vi "main.vi"(7 "Last Experiment of the Day":bool, 8 "error in":errorcluster, 9 "SSH password":string, 10 "SSH user name":string, 11 "Tags":string) -> (0 "error out":errorcluster)   [LabVIEW 2019]
uses:
  WormTrackSnippetCluster.ctl
  TrackTerminationReasonEnum.ctl
  HeadTailContinuousGWN.lvclass
  C:/github/ProjectAPI/LabviewVIs/StimulusObject.lvclass
  HeadTailContinuousGWNClass/HeadTailContinuousGWNInputCluster.ctl
  <vilib>/vision/driver/IMAQdx.llb/IMAQdx Acquisition Mode.ctl
  CompletedTracksFunctionalGlobalOperations.ctl
  ActiveTracksFunctionalGlobalOperations.ctl
  TimestampsFunctionalGlobalOperations.ctl
  <vilib>/vision/driver/IMAQdx.llb/IMAQdx Buffer Number Mode.ctl
  center2rectangle.vi
  overlay_crossmarks.vi
  ParametersGlobal.vi
  DebugGlobal.vi
  <vilib>/vision/driver/NI_Vision_Acquisition_Software.lvlib
  <vilib>/vision/NI_Vision_Development_Module.lvlib
panel:
  out "Experiment Start":dbl
  out "Spatial Correction Fit Error (camera pixel)":dbl
  out "transformation_description":dbl[](array[numeric])
  out "Latest Active Worm Tracks":T1[](array[typedef])
  out "Mature Tracks Count":i32
  out "Active Tracks Count":i32
  out "total time elapsed (s)":dbl
  out "Draw Stimulus Missed Frames":dbl
  out "Tracking Missed Frames":dbl
  out "Camera Missed Frames":dbl
  out "Last Calibration":dbl
  in  "GUI Refresh Period (ms)":u32=10000
  out "Stop Debug":string
  out "Completed Tracks #":i32
  out "Projector Saving Lag (Projector Frames)":i32
  out "Stimulus Image":T3(plugin-control)
  out "Closed Loop Lag (frames)":i32
  out "Single Worm Image":T3(plugin-control)
  in  "Selected Track Index":i32
  out "Tracking Rate (Hz)":dbl
  out "Last Median Filter Updated":string
  out "median closed loop lag (ms)":dbl
  out "Draw Stimulus Frame Rate (Hz)":dbl
  out "Saving Lag (Camera Frames)":i32
  out "Camera Frame Rate (Hz)":dbl
  out "Camera Buffer Number":u32
  in  "stop":bool
  out "Camera Input":T3(plugin-control)
  out "Processed Image":T3(plugin-control)
  # "Max Spatial Drift (mm) Since:"
  # "Guide to spatial re-alignment Processed Image:\nPink circles represents previous calibration locations.\nAqua circle means the calibration for this iteration.\nYellow lines show deviation from previous calibration loation to locations extracted just now.\nMagenta lines at the end shows drift since the experiment began"
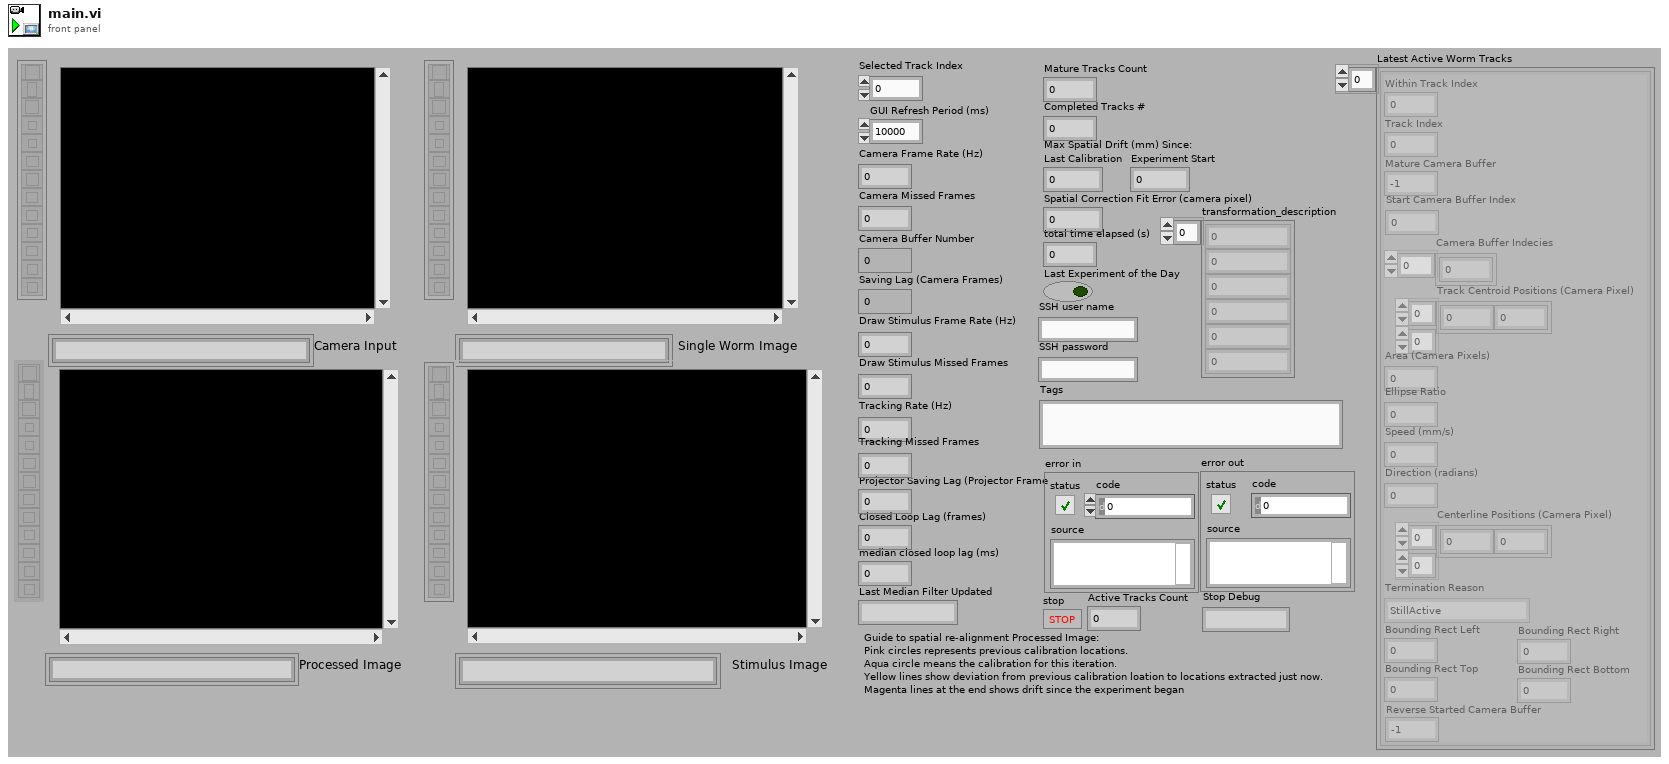
[diagram p1: front panel]
types:
  T1 = typedef "WormTrackSnippetCluster.ctl" = cluster{"Track Centroid Positions (Camera Pixel)":sgl[][], "Within Track Index":i32, "Camera Buffer Indecies":i32[], "Area (Camera Pixels)":i32, "Speed (mm/s)":sgl, "Direction (radians)":sgl, "Centerline Positions (Camera Pixel)":sgl[][], "Ellipse Ratio":sgl, "Termination Reason":T2, "Track Index":i32, "Bounding Rect Left":i32, "Bounding Rect Top":i32, "Bounding Rect Right":i32, "Bounding Rect Bottom":i32, "Mature Camera Buffer":i32, "Start Camera Buffer Index":i32, "Reverse Started Camera Buffer":i32}
  T2 = typedef "TrackTerminationReasonEnum.ctl" = enum16{"StillActive", "MaxDisplacement", "NoBlobsLeft", "AreaIncrease", "AreaDecrease", "ExperimentEnded"}
  T3 = typedef "IMAQ Image.ctl" = refnum<image>
  T4 = typedef "HeadTailContinuousGWN.lvclass/HeadTailContinuousGWNInputCluster.ctl" = cluster{"offset (red uW/mm^2m, blue is negative)":sgl, "correlation time (s)":sgl, "standard deviation (red uW/mm^2)":sgl, "Max blue stimulus (uW/mm^2)":sgl, "Max red stimulus (uW/mm^2)":sgl, "dot radius (mm)":sgl}
  T5 = typedef "TimestampsFunctionalGlobalOperations.ctl" = enum16{"Initialize", "Dump", "UpdateTime", "ReadTime"}
  T6 = typedef "ActiveTracksFunctionalGlobalOperations.ctl" = enum16{"Initialize", "ReadFullTrackGivenWormIndex", "WriteFullTrack", "ReadTrackSnippets", "WriteTrackGivenSnippets", "ReadStimulusSnippets", "StartNewTracksGivenSnippets", "EndTracksGivenSnippets", "WriteStimulusObjectGivenWormIndex", "CompleteAllActiveTracks", "ReturnAllActiveTrackIndecies"}
  T7 = typedef "CompletedTracksFunctionalGlobalOperations.ctl" = enum16{"Initialize", "ReturnAllTracks", "ReturnLastIndex", "SaveCompletedTracks", "TrimAndReturnAllTracks"}
  T8 = typedef "NI_Vision_Acquisition_Software.lvlib/IMAQdx Buffer Number Mode.ctl" = enum32{"Next", "Last", "Buffer Number", "Every", "Last New"}
  T9 = typedef "Image Type" = u32
  T10 = typedef "NI_Vision_Acquisition_Software.lvlib/IMAQdx Acquisition Mode.ctl" = enum32{"One Shot", "Continuous"}
  T11 = typedef "IMAQdx.ctl" = refnum<k21>
  T12 = typedef "WormTrackCluster.ctl" = cluster{"Track Centroid Positions (Camera Pixel)":sgl[][], "Within Track Index":i32, "Camera Buffer Indecies":i32[], "Area (Camera Pixels)":i32[], "Speed (mm/s)":sgl[], "Direction (radians)":sgl[], "Centerline Positions (Camera Pixel)":sgl[][][], "Ellipse Ratio":sgl[], "Stimulus Object":refnum<class "StimulusObject.lvclass">, "Termination Reason":T2, "Track Index":i32, "Mature Camera Buffer":i32, "Reverse Started Camera Buffer":i32}
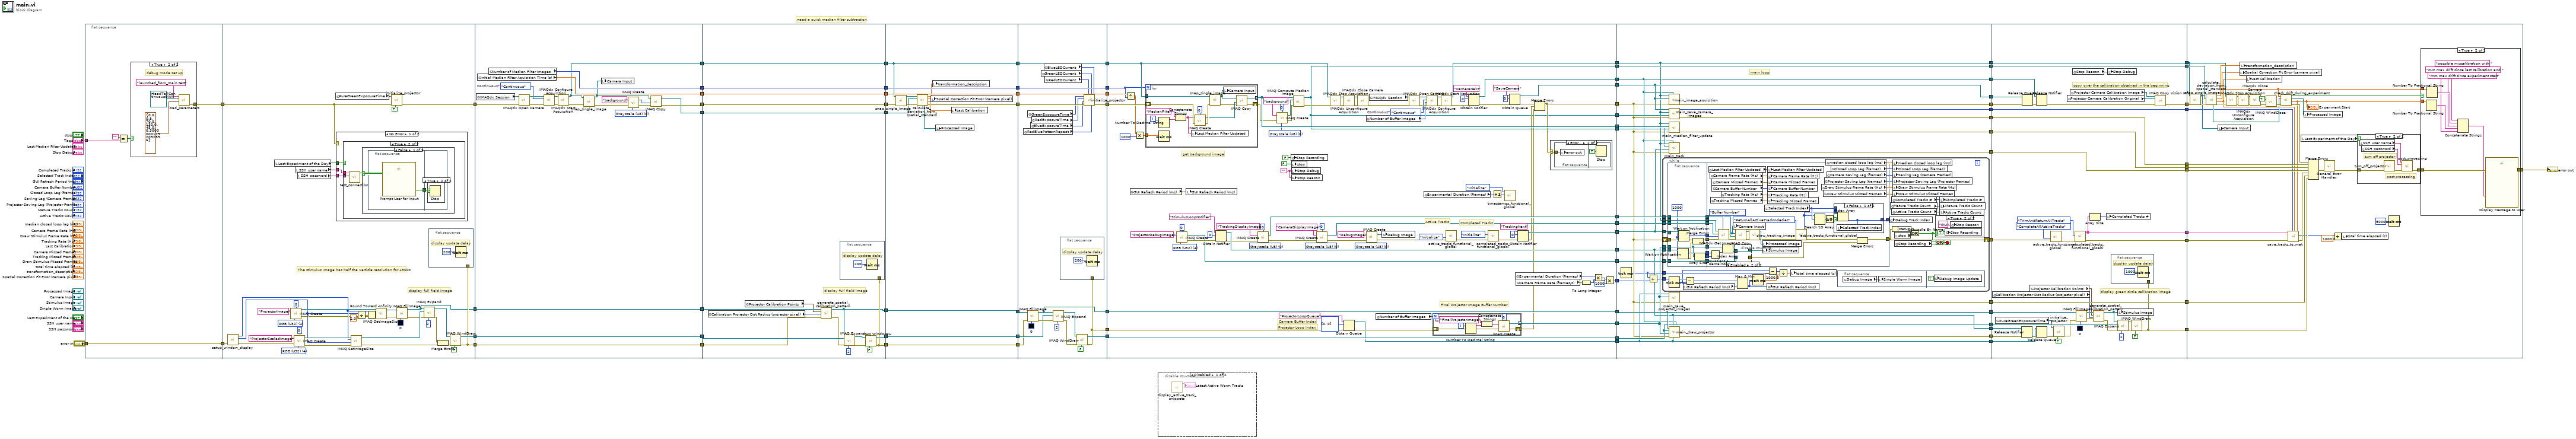
[diagram p0: block diagram]
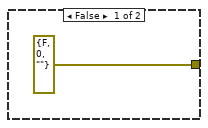
[diagram p3: hidden frame]
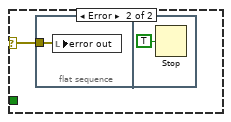
[diagram p7: hidden frame]
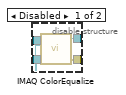
[diagram p11: hidden frame]
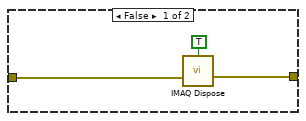
[diagram p12: hidden frame]
diagram:
  # "need a quick median filter subtraction"
  n1 = flat-sequence {
    tunnel: "Tags" -> [w85]
    tunnel: "error in" -> [w89]
    tunnel: [w89] -> w28
    tunnel: [w86] -> w27
    tunnel: [w125] -> w77
    tunnel: [w104] -> w76
    tunnel: [w99] -> w75
    tunnel: [w97] -> w63
    tunnel: w28 -> [w113]
    tunnel: w27 -> [w98]
    tunnel: [w148] -> w20
    tunnel: w77 -> [w157]
    tunnel: w76 -> [w158]
    tunnel: [w158] -> w21
    tunnel: [w154] -> w22
    tunnel: w75 -> [w156]
    tunnel: [w167] -> w23
    tunnel: [w166] -> w24
    tunnel: w63 -> [w160]
    tunnel: [w157] -> w25
    tunnel: [w156] -> w26
    tunnel: [w147] -> w4
    tunnel: w26 -> [w173]
    tunnel: [w168] -> w19
    tunnel: w25 -> [w179]
    tunnel: [w178] -> w17
    tunnel: w24 -> [w185]
    tunnel: [w185] -> w15
    tunnel: w23 -> [w184]
    tunnel: [w184] -> w13
    tunnel: w22 -> [w183]
    tunnel: [w183] -> w11
    tunnel: w21 -> [w174]
    tunnel: [w175] -> w9
    tunnel: w20 -> [w182]
    tunnel: [w182] -> w7
    tunnel: [w176] -> w5
    tunnel: w4 -> [w176]
    tunnel: w19 -> [w201]
    tunnel: [w201] -> w18
    tunnel: w17 -> [w200]
    tunnel: [w200] -> w16
    tunnel: w15 -> [w199]
    tunnel: [w199] -> w14
    tunnel: w13 -> [w198]
    tunnel: [w198] -> w12
    tunnel: w11 -> [w193]
    tunnel: [w193] -> w10
    tunnel: w9 -> [w197]
    tunnel: [w197] -> w8
    tunnel: w7 -> [w195]
    tunnel: [w187] -> w6
    tunnel: w5 -> [w191]
    tunnel: [w209] -> w35
    tunnel: [w225] -> w34
    tunnel: [w224] -> w33
    tunnel: [w223] -> w32
    tunnel: [w222] -> w31
    tunnel: [w221] -> w30
    tunnel: [w220] -> w29
    tunnel: w18 -> [w214]
    tunnel: w16 -> [w213]
    tunnel: w14 -> [w220]
    tunnel: w12 -> [w221]
    tunnel: w10 -> [w223]
    tunnel: w8 -> [w212]
    tunnel: w6 -> [w210]
    tunnel: [w303] -> w84
    tunnel: [w252] -> w83
    tunnel: [w291] -> w82
    tunnel: [w240] -> w81
    tunnel: w35 -> [w316]
    tunnel: w34 -> [w303]
    tunnel: w33 -> [w246]
    tunnel: w32 -> [w263]
    tunnel: w31 -> [w291]
    tunnel: [w227] -> w80
    tunnel: [w312] -> w79
    tunnel: [w311] -> w78
    tunnel: [w308] -> w74
    tunnel: [w292] -> w73
    tunnel: [w286] -> w72
    tunnel: [w283] -> w71
    tunnel: [w278] -> w70
    tunnel: [w275] -> w69
    tunnel: [w268] -> w68
    tunnel: w30 -> [w251]
    tunnel: w29 -> [w250]
    tunnel: [w227] -> w64
    tunnel: [w227] -> w62
    tunnel: [w244] -> w37
    tunnel: [w236] -> w36
    tunnel: [w372] -> w61
    tunnel: w84 -> [w357]
    tunnel: w83 -> [w352]
    tunnel: w82 -> [w358]
    tunnel: w81 -> [w348]
    tunnel: [w353] -> w60
    tunnel: [w371] -> w59
    tunnel: [w370] -> w58
    tunnel: [w352] -> w56
    tunnel: w80 -> [w351]
    tunnel: w79 -> [w368]
    tunnel: [w369] -> w54
    tunnel: w78 -> [w353]
    tunnel: w74 -> [w349]
    tunnel: [w349] -> w52
    tunnel: [w367] -> w51
    tunnel: w73 -> [w366]
    tunnel: [w365] -> w49
    tunnel: w72 -> [w355]
    tunnel: w71 -> [w354]
    tunnel: w70 -> [w356]
    tunnel: w69 -> [w364]
    tunnel: w68 -> [w363]
    tunnel: [w362] -> w48
    tunnel: [w356] -> w46
    tunnel: w64 -> [w361]
    tunnel: [w360] -> w45
    tunnel: w62 -> [w359]
    tunnel: [w359] -> w44
    tunnel: [w357] -> w40
    tunnel: [w358] -> w39
    tunnel: [w354] -> w38
    tunnel: w37 -> [w350]
    tunnel: w36 -> [w346]
    tunnel: w61 -> [w505]
    tunnel: w60 -> [w513]
    tunnel: w59 -> [w511]
    tunnel: w58 -> [w520]
    tunnel: [w520] -> w57
    tunnel: w56 -> [w519]
    tunnel: [w519] -> w55
    tunnel: w54 -> [w518]
    tunnel: [w518] -> w53
    tunnel: w52 -> [w512]
    tunnel: w51 -> [w517]
    tunnel: [w517] -> w50
    tunnel: w49 -> [w507]
    tunnel: w48 -> [w516]
    tunnel: [w516] -> w47
    tunnel: w46 -> [w504]
    tunnel: w45 -> [w482]
    tunnel: w44 -> [w515]
    tunnel: [w515] -> w43
    tunnel: [w485] -> w42
    tunnel: [w492] -> w41
    tunnel: w40 -> [w499]
    tunnel: w39 -> [w495]
    tunnel: w38 -> [w493]
    tunnel: [w482] -> w3
    tunnel: [w481] -> w2
    tunnel: [w480] -> w1
    tunnel: w57 -> [w553]
    tunnel: w55 -> [w538]
    tunnel: w53 -> [w555]
    tunnel: w50 -> [w556]
    tunnel: w47 -> [w554]
    tunnel: [w548] -> w66
    tunnel: w43 -> [w541]
    tunnel: w42 -> [w542]
    tunnel: w41 -> [w547]
    tunnel: w3 -> [w528]
    tunnel: w2 -> [w527]
    tunnel: w1 -> [w526]
    frame #0 {
      n2 = Equal?(x="", y=w85) -> (x = y?=w88:bool)
      n3 = case shown="True" w88 {
        tunnel: [errorcluster {"status"=FALSE, "code"=0, "source"=""} ("error in") w94] -> w86
        frame False {
        }
        frame True {
          # "debug mode set up"
          n4 = call "load_parameters.vi"("StimulusObject Parameters"=T4 {"offset (red uW/mm^2m, blue is negative)"=0.0, "correlation time (s)"=0.5, "standard deviation (red uW/mm^2)"=70.0, "Max blue stimulus (uW/mm^2)"=130.0, "Max red stimulus (uW/mm^2)"=45.0, "dot radius (mm)"=0.3} ("HeadTailContinousGWNInputCluser"), "StimulusObjectClassInput"=refnum<class "HeadTailContinuousGWN.lvclass"> refnum ("HeadTailContinuousGWN.lvclass"), "Tags"="launched_from_main test") -> ("error out"=w94:errorcluster)  [unwired: 6 in, 2 out]
        }
      }
    }
    frame #1 {
      w123 = T9 4 items=["Grayscale (U8)", "Grayscale (I16)", "Grayscale (SGL)", "Complex (CSG)", "RGB (U32)", "HSL (U32)", "RGB (U64)"] ("Image Type")
      w127 = T9 4 items=["Grayscale (U8)", "Grayscale (I16)", "Grayscale (SGL)", "Complex (CSG)", "RGB (U32)", "HSL (U32)", "RGB (U64)"] ("Image Type")
      # "The stimulus Image has half the verticle resolution for 4500s"
      # "display full field image"
      n5 = call "setup_window_display.vi"("error in (no error)"=w113) -> ("error out"=w130:errorcluster, "Height"=w117:i16, "Width"=w121:i16)  [unwired: 8 in]
      n6 = local read "Last Experiment of the Day"() -> (w110:bool)
      n7 = call "IMAQ Create"("Border Size"=0, "Image Name"="ProjectorImage", "Image Type"=w123) -> ("New Image"=w122:T3, "error out"=w116:errorcluster)  [unwired: 2 in]
      n8 = call "IMAQ Create"("Border Size"=0, "Image Name"="ProjectorScaledImage", "Image Type"=w127, "error in (no error)"=w130) -> ("New Image"=w131:T3, "error out"=w132:errorcluster)  [unwired: 1 in]
      n9 = local read "SSH user name"() -> (w111:string)
      n10 = local read "SSH password"() -> (w112:string)
      n11 = global read "ParametersGlobal.vi" "PureGreenExposureTime"() -> (w95:i32)
      n12 = case shown="No Error" w98 {
        selector: w98 -> [_ w143]
        tunnel: w112 -> [w136 _]
        tunnel: w111 -> [w135 _]
        tunnel: w110 -> [w134 _]
        frame No Error {
          n13 = case shown="True" w134 {
            tunnel: w136 -> [_ w139]
            tunnel: w135 -> [_ w137]
            frame False {
            }
            frame True {
              n14 = call "test_connection.vi"("Username"=w137, "Password"=w139) -> ("Connection Successful"=w138:bool)  [unwired: 7 in]
              n15 = case shown="False" w138 {
                frame False {
                  n16 = flat-sequence {
                    tunnel: [w141] -> w140
                    tunnel: w140 -> [w142]
                    frame #0 {
                      n17 = call "Prompt User for Input"() -> ("OK"=w141:bool)  [unwired: 18 in, 1 out]
                    }
                    frame #1 {
                      n18 = case shown="True" w142 {
                        frame False {
                        }
                        frame True {
                          n19 = Stop() -> ()  [unwired: 1 in]
                        }
                      }
                    }
                  }
                }
                frame True {
                }
              }
            }
          }
        }
        frame Error {
          n20 = flat-sequence {
            tunnel: w143 -> [w144]
            frame #0 {
              n21 = local write "error out"(w144) -> ()
            }
            frame #1 {
              n22 = Stop(stop? (T)=TRUE) -> ()
            }
          }
        }
      }
      n23 = call "IMAQ SetImageSize"("error in (no error)"=w132, "Y Resolution"=w117, "X Resolution"=w121, "Image"=w131) -> ("error out"=w105:errorcluster, "Image Out"=w108:T3)  [unwired: 1 in]
      n24 = Divide(x=w117, y=2.0) -> (x/y=w119:dbl)
      n25 = Round Toward -Infinity(1:w119) -> (0:w120:dbl)
      n26 = call "IMAQ SetImageSize"("error in (no error)"=w116, "Y Resolution"=w120, "X Resolution"=w121, "Image"=w122) -> ("error out"=w102:errorcluster, "Image Out"=w100:T3)  [unwired: 1 in]
      n27 = call "initialize_projector.vi"("Green Only"=TRUE, "error in"=w98, "green exp_time_us"=w95) -> ("error out"=w97:errorcluster)  [unwired: 8 in]
      n28 = call "IMAQ FillImage"("Color Pixel Value"=u32 0, "error in (no error)"=w102, "Image"=w100) -> ("error out"=w101:errorcluster, "Image Out"=w99:T3)  [unwired: 7 in]
      n29 = call "IMAQ Expand"("Y Duplication Step"=2, "error in (no error)"=w101, "Image Dst"=w108, "Image Src"=w99) -> ("error out"=w106:errorcluster, "Image Dst Out"=w107:T3)  [unwired: 6 in]
      n30 = flat-sequence {
        tunnel: w104 -> [_]
        frame #0 {
          # "display update delay"
          n31 = Wait (ms)(milliseconds to wait=u32 200) -> ()  [unwired: 1 out]
        }
      }
      n32 = Merge Errors(w106, w105) -> (w115:errorcluster)
      n33 = call "IMAQ WindDraw"("Resize to Image Size? (Y)"=FALSE, "error in (no error)"=w115, "Image"=w107) -> ("error out"=w104:errorcluster, "Image Out (duplicate)"=w125:T3)  [unwired: 7 in]
    }
    frame #2 {
      w146 = T9 0 items=["Grayscale (U8)", "Grayscale (I16)", "Grayscale (SGL)", "Complex (CSG)", "RGB (U32)", "HSL (U32)", "RGB (U64)", "Grayscale (U16)"] ("Image Type")
      w159 = IMAQdx_Acquisition_Mode."Continuous"  # Continuous?
      n34 = global read "ParametersGlobal.vi" "IMAQdx Session"() -> (w165:T11)
      n35 = global read "ParametersGlobal.vi" "Initial Median Filter Aquisition Time (s)"() -> (w167:dbl)
      n36 = global read "ParametersGlobal.vi" "Number of Median Filter Images"() -> (w166:i32)
      n37 = call <vilib>:"IMAQdx Open Camera.vi"("error in"=w160, "Session In"=w165) -> ("error out"=w162:errorcluster, "Session Out"=w161:T11)  [unwired: 8 in]
      n38 = call <vilib>:"IMAQdx Configure Acquisition.vi"("error in"=w162, "Continuous?"=w159, "Session In"=w161) -> ("error out"=w163:errorcluster, "Session Out"=w164:T11)  [unwired: 7 in]
      n39 = call <vilib>:"IMAQdx Start Acquisition.vi"("error in"=w163, "Session In"=w164) -> ("error out"=w155:errorcluster, "Session Out"=w154:T11)  [unwired: 8 in]
      n40 = call "snap_single_image.vi"("error in (no error)"=w155, "Session In"=w154) -> ("error out"=w152:errorcluster, "Image Out"=w149:T3)  [unwired: 8 in]
      n41 = local write "Camera Input"(w149) -> ()
      n42 = call "IMAQ Create"("Image Name"="background", "Image Type"=w146, "error in (no error)"=w152) -> ("New Image"=w150:T3, "error out"=w151:errorcluster)  [unwired: 2 in]
      n43 = call "IMAQ Copy"("error in (no error)"=w151, "Image Dst"=w150, "Image Src"=w149) -> ("error out"=w148:errorcluster, "Image Dst Out"=w147:T3)  [unwired: 3 in]
    }
    frame #3 {
      # "display full field image"
      n44 = global read "ParametersGlobal.vi" "Calibration Projector Dot Radius (projector pixel)"() -> (w171:i32)
      n45 = global read "ParametersGlobal.vi" "Projector Calibration Points"() -> (w170:cluster{"X":dbl, "Y":dbl}[])
      n46 = call "generate_spatial_calibration_pattern.vi"("error in (no error)"=w174, "Dot Radius (Projector Pixels)"=w171, "Points Array"=w170, "StimulusImageIn"=w173) -> ("error out"=w172:errorcluster, "StimulusImageOut"=w168:T3)  [unwired: 6 in]
      n47 = flat-sequence {
        tunnel: w175 -> [_]
        frame #0 {
          # "display update delay"
          n48 = Wait (ms)(milliseconds to wait=u32 200) -> ()  [unwired: 1 out]
        }
      }
      n49 = call "IMAQ Expand"("Y Duplication Step"=2, "error in (no error)"=w172, "Image Dst"=w179, "Image Src"=w168) -> ("error out"=w177:errorcluster, "Image Dst Out"=w169:T3)  [unwired: 6 in]
      n50 = call "IMAQ WindDraw"("Resize to Image Size? (Y)"=FALSE, "error in (no error)"=w177, "Image"=w169) -> ("error out"=w175:errorcluster, "Image Out (duplicate)"=w178:T3)  [unwired: 7 in]
    }
    frame #4 {
      n51 = call "snap_single_image.vi"("error in (no error)"=w195, "Session In"=w193) -> ("error out"=w194:errorcluster, "Image Out"=w192:T3)  [unwired: 8 in]
      n52 = call "calculate_deviation_from_spatial_standard.vi"("Image Src"=w192, "Background Image"=w191, "error in (no error)"=w194) -> ("Processed Image"=w188:T3, "transformation_description"=w196:dbl[], "fit least squares error (camera pixel)"=w189:dbl, "max spatial drift (mm)"=w190:dbl, "error out"=w187:errorcluster)  [unwired: 3 in]
      n53 = local write "Spatial Correction Fit Error (camera pixel)"(w189) -> ()
      n54 = local write "transformation_description"(w196) -> ()
      n55 = local write "Processed Image"(w188) -> ()
      n56 = local write "Last Calibration"(w190) -> ()
    }
    frame #5 {
      n57 = global read "ParametersGlobal.vi" "RedBluePatternRepeat"() -> (w202:i32)
      n58 = call "IMAQ FillImage"("Color Pixel Value"=u32 0, "error in (no error)"=w212, "Image"=w214) -> ("error out"=w219:errorcluster, "Image Out"=w222:T3)  [unwired: 7 in]
      n59 = global read "ParametersGlobal.vi" "GreenExposureTime"() -> (w205:i32)
      n60 = global read "ParametersGlobal.vi" "BlueExposureTime"() -> (w203:i32)
      n61 = global read "ParametersGlobal.vi" "RedExposureTime"() -> (w204:i32)
      n62 = global read "ParametersGlobal.vi" "GreenLEDCurrent"() -> (w207:u8)
      n63 = global read "ParametersGlobal.vi" "BlueLEDCurrent"() -> (w206:u8)
      n64 = global read "ParametersGlobal.vi" "RedLEDCurrent"() -> (w208:u8)
      n65 = call "IMAQ Expand"("Y Duplication Step"=2, "error in (no error)"=w219, "Image Dst"=w213, "Image Src"=w222) -> ("error out"=w215:errorcluster, "Image Dst Out"=w211:T3)  [unwired: 6 in]
      n66 = flat-sequence {
        tunnel: w224 -> [_]
        frame #0 {
          # "display update delay"
          n67 = Wait (ms)(milliseconds to wait=u32 200) -> ()  [unwired: 1 out]
        }
      }
      n68 = call "IMAQ WindDraw"("Resize to Image Size? (Y)"=FALSE, "error in (no error)"=w215, "Image"=w211) -> ("error out"=w224:errorcluster, "Image Out (duplicate)"=w225:T3)  [unwired: 7 in]
      n69 = call "initialize_projector.vi"("BlueCurrent"=w206, "RedBluePatternRepeat"=w202, "GreenCurrent"=w207, "RedCurrent"=w208, "error in"=w210, "blue exp_time_us"=w203, "red exp_time_us"=w204, "green exp_time_us"=w205) -> ("error out"=w209:errorcluster)  [unwired: 3 in]
    }
    frame #6 {
      w229 = T9 0 items=["Grayscale (U8)", "Grayscale (I16)", "Grayscale (SGL)", "Complex (CSG)", "RGB (U32)", "HSL (U32)", "RGB (U64)", "Grayscale (U16)"] ("Image Type")
      w258 = IMAQdx_Acquisition_Mode."Continuous"  # Continuous?
      w247 = ""
      w272 = T9 0 items=["Grayscale (U8)", "Grayscale (I16)", "Grayscale (SGL)", "Complex (CSG)", "RGB (U32)", "HSL (U32)", "RGB (U64)", "Grayscale (U16)"] ("Image Type")
      w282 = T9 4 items=["Grayscale (U8)", "Grayscale (I16)", "Grayscale (SGL)", "Complex (CSG)", "RGB (U32)", "HSL (U32)", "RGB (U64)", "Grayscale (U16)"] ("Image Type")
      w296 = T9 0 items=["Grayscale (U8)", "Grayscale (I16)", "Grayscale (SGL)", "Complex (CSG)", "RGB (U32)", "HSL (U32)", "RGB (U64)", "Grayscale (U16)"] ("Image Type")
      w301 = T9 0 items=["Grayscale (U8)", "Grayscale (I16)", "Grayscale (SGL)", "Complex (CSG)", "RGB (U32)", "HSL (U32)", "RGB (U64)", "Grayscale (U16)"] ("Image Type")
      # "Projector Loop Index"
      # "Camera Buffer Index"
      # "Final Projector Image Buffer Number"
      # "Active Tracks"
      # "Completed Tracks"
      # "get background image"
      n70 = Divide(x=w251, y=w250) -> (x/y=w307:dbl)
      n71 = global read "DebugGlobal.vi" "GUI Refresh Period (ms)"() -> (w233:u32)
      n72 = Multiply(x=w307, y=1000) -> (x*y=w305:dbl)
      n73 = for {
        N: w250 -> [_]
        tunnel: w263 -> [w344]
        shift-right: [w333] -> w302
        shift-left: w316 -> [w340]
        tunnel: [w336] -> w312 mode=indexing
        tunnel: w305 -> [w335]
        i -> [w343]
        n74 = Wait (ms)(milliseconds to wait=w335) -> ()  [unwired: 1 out]
        n75 = Number To Decimal String(number=w343) -> (decimal integer string=w342:string)  [unwired: 1 in]
        n76 = Concatenate Strings("MedianFilter", w342) -> (w331:string)
        n77 = local write "Last Median Filter Updated"(w331) -> ()
        n78 = call "IMAQ Create"("Border Size"=0, "Image Name"=w331, "error in (no error)"=w340) -> ("New Image"=w338:T3, "error out"=w339:errorcluster)  [unwired: 2 in]
        n79 = call "snap_single_image.vi"("error in (no error)"=w339, "Session In"=w344) -> ("error out"=w337:errorcluster, "Image Out"=w332:T3)  [unwired: 8 in]
        n80 = local write "Camera Input"(w332) -> ()
        n81 = call "IMAQ Copy"("error in (no error)"=w337, "Image Dst"=w338, "Image Src"=w332) -> ("error out"=w333:errorcluster, "Image Dst Out"=w336:T3)  [unwired: 3 in]
      }
      n82 = call "IMAQ Create"("Border Size"=0, "Image Name"="ProjectorDebugImage", "Image Type"=w282) -> ("New Image"=w275:T3, "error out"=w276:errorcluster)  [unwired: 2 in]
      n83 = local write "GUI Refresh Period (ms)"(w233) -> ()
      n84 = Obtain Notifier(name (unnamed)="StimulusLoopNotifier", notification data type=0, error in (no error)=w276) -> (notifier out=w278:refnum<notifier>, error out=w270:errorcluster)  [unwired: 1 in, 1 out]
      n85 = call "IMAQ Create"("Border Size"=0, "Image Name"="TrackingDisplayImage", "Image Type"=w272, "error in (no error)"=w270) -> ("New Image"=w268:T3, "error out"=w269:errorcluster)  [unwired: 1 in]
      n86 = call "IMAQ Create"("Border Size"=0, "Image Name"="background", "Image Type"=w229, "error in (no error)"=w302) -> ("New Image"=w313:T3, "error out"=w314:errorcluster)  [unwired: 1 in]
      n87 = global write "DebugGlobal.vi" "Stop Recording"(FALSE ("Stop Recording")) -> ()
      n88 = local write "stop"(FALSE) -> ()
      n89 = local write "Stop Debug"(w247) -> ()
      n90 = global write "DebugGlobal.vi" "Stop Reason"(w247) -> ()
      n91 = call "IMAQ Compute Median Image"("error in (no error)"=w314, "Image Dst"=w313, "Images"=w312) -> ("error out"=w228:errorcluster, "Image Dst Out"=w227:T3)  [unwired: 7 in]
      n92 = call "IMAQ Create"("Border Size"=0, "Image Name"="CameraDisplayImage", "Image Type"=w296, "error in (no error)"=w269) -> ("New Image"=w292:T3, "error out"=w293:errorcluster)  [unwired: 1 in]
      n93 = call <vilib>:"IMAQdx Stop Acquisition.vi"("error in"=w228, "Session In"=w263) -> ("error out"=w264:errorcluster, "Session Out"=w265:T11)  [unwired: 8 in]
      n94 = call <vilib>:"IMAQdx Unconfigure Acquisition.vi"("error in"=w264, "Session In"=w265) -> ("error out"=w267:errorcluster, "Session Out"=w266:T11)  [unwired: 8 in]
      n95 = Obtain Queue(name (unnamed)="ProjectorLoopQueue", element data type=i32[] [0, 0], error in (no error)=w246) -> (queue out=w283:refnum<queue>, error out=w284:errorcluster)  [unwired: 2 in, 1 out]
      n96 = call <vilib>:"IMAQdx Close Camera.vi"("error in"=w267, "Session In"=w266) -> ("error out"=w256:errorcluster)  [unwired: 9 in]
      n97 = global read "ParametersGlobal.vi" "Number of Buffer Images"() -> (w254:i32)
      n98 = call "IMAQ Create"("Image Name"="DebugImage", "Image Type"=w301, "error in (no error)"=w293) -> ("New Image"=w299:T3, "error out"=w245:errorcluster)  [unwired: 2 in]
      n99 = global read "ParametersGlobal.vi" "IMAQdx Session"() -> (w257:T11)
      n100 = global read "ParametersGlobal.vi" "Number of Buffer Images"() -> (w253:i32)
      n101 = global write "DebugGlobal.vi" "Debug Image"(w299) -> ()
      n102 = call <vilib>:"IMAQdx Open Camera.vi"("error in"=w256, "Session In"=w257) -> ("error out"=w261:errorcluster, "Session Out"=w262:T11)  [unwired: 8 in]
      n103 = global read "ParametersGlobal.vi" "Experimental Duration (Frames)"() -> (w232:i32)
      n104 = call <vilib>:"IMAQdx Configure Acquisition.vi"("error in"=w261, "Number of Buffers"=w254, "Continuous?"=w258, "Session In"=w262) -> ("error out"=w260:errorcluster, "Session Out"=w259:T11)  [unwired: 6 in]
      n105 = for {
        N: w253 -> [_]
        shift-right: [w324] -> w241
        shift-left: w284 -> [w327]
        tunnel: [w323] -> w286 mode=indexing
        i -> [w330]
        n106 = Number To Decimal String(number=w330) -> (decimal integer string=w329:string)  [unwired: 1 in]
        n107 = Concatenate Strings("FinalProjectorImage", w329) -> (w326:string)
        n108 = call "IMAQ Create"("Border Size"=0, "Image Name"=w326, "error in (no error)"=w327) -> ("New Image"=w323:T3, "error out"=w324:errorcluster)  [unwired: 2 in]
      }
      n109 = call <vilib>:"IMAQdx Start Acquisition.vi"("error in"=w260, "Session In"=w259) -> ("error out"=w255:errorcluster, "Session Out"=w252:T11)  [unwired: 8 in]
      n110 = call "active_tracks_functional_global.vi"("error in"=w245, "Operations"=ActiveTracksFunctionalGlobalOperations."Initialize") -> ("error out"=w288:errorcluster)  [unwired: 5 in, 4 out]
      n111 = Obtain Notifier(name (unnamed)="CameraNext", notification data type=u32 0, error in (no error)=w255) -> (notifier out=w308:refnum<notifier>, error out=w249:errorcluster)  [unwired: 1 in, 1 out]
      n112 = call "completed_tracks_functional_gloabl.vi"("error in (no error)"=w288, 10:CompletedTracksFunctionalGlobalOperations."Initialize") -> ("error out"=w289:errorcluster)  [unwired: 6 in, 3 out]
      n113 = Increment(x=w232) -> (x+1=w231:i32)
      n114 = call "timestamps_functional_global.vi"("Buffer Number"=w231, "Operation"=TimestampsFunctionalGlobalOperations."Initialize") -> ()  [unwired: 3 in, 3 out]
      n115 = Obtain Queue(name (unnamed)="SaveCamera", element data type=u32 0, error in (no error)=w249) -> (queue out=w311:refnum<queue>, error out=w243:errorcluster)  [unwired: 2 in, 1 out]
      n116 = global read "ParametersGlobal.vi" "Experimental Duration (Frames)"() -> (w239:i32)
      n117 = global read "ParametersGlobal.vi" "Camera Frame Rate (frames/s)"() -> (w235:sgl)
      n118 = Obtain Notifier(name (unnamed)="TrackingNext", notification data type=u32 0, error in (no error)=w289) -> (notifier out=w244:refnum<notifier>, error out=w242:errorcluster)  [unwired: 1 in, 1 out]
      n119 = Merge Errors(w243, w242, w241) -> (w240:errorcluster)
      n120 = case shown="Error .." w240 {
        selector: w240 -> [_ w320]
        frame No Error {
        }
        frame Error {
          n121 = flat-sequence {
            tunnel: w320 -> [w321]
            frame #0 {
              n122 = local write "error out"(w321) -> ()
            }
            frame #1 {
              n123 = Stop(stop? (T)=TRUE) -> ()
            }
          }
        }
      }
      n124 = To Long Integer(number=w235) -> (32bit integer=w234:i32)
      n125 = Multiply(x=w239, y=w234) -> (x*y=w238:i32)
      n126 = Multiply(x=w238, y=1000) -> (x*y=w236:i32)
    }
    frame #7 {
      # "main loop"
      n127 = Tick Count (ms)() -> (millisecond timer value=w347:u32)
      n128 = Add(x=w347, y=w346) -> (x+y=w345:u32)
      n129 = while {
        shift-right: [w406] -> w365
        shift-left: w348 -> [w413]
        tunnel: w350 -> [w414]
        tunnel: w352 -> [w410]
        tunnel: w366 -> [w407]
        tunnel: w356 -> [w404]
        tunnel: w355 -> [w402]
        tunnel: w364 -> [w400]
        tunnel: w363 -> [w397]
        tunnel: w347 -> [w387]
        tunnel: w345 -> [w382]
        stop <- w390 stop-if-true
        n130 = flat-sequence {
          tunnel: w414 -> [w433]
          tunnel: w413 -> [w432]
          tunnel: [w426] -> w412
          tunnel: [w431] -> w411
          tunnel: w410 -> [w430]
          tunnel: [w430] -> w409
          tunnel: [w429] -> w408
          tunnel: w407 -> [w429]
          tunnel: w404 -> [w428]
          tunnel: [w427] -> w403
          tunnel: w402 -> [w419]
          tunnel: [w419] -> w401
          tunnel: w400 -> [w423]
          tunnel: [w423] -> w399
          tunnel: [w422] -> w398
          tunnel: w397 -> [w422]
          tunnel: [w420] -> w388
          tunnel: w412 -> [w466]
          tunnel: [w452] -> w406
          tunnel: w411 -> [w465]
          tunnel: w409 -> [w464]
          tunnel: w408 -> [w463]
          tunnel: w403 -> [w462]
          tunnel: w401 -> [w461]
          tunnel: w399 -> [w459]
          tunnel: w398 -> [w456]
          tunnel: w388 -> [w443]
          tunnel: [w436] -> w375
          frame #0 {
            w421 = 1000 ("timeout in ms (-1)")
            n131 = Wait on Notification(notifier=w428, timeout in ms (-1)=w421) -> (notification=w427:i32, error out=w424:errorcluster)  [unwired: 2 in, 2 out]
            n132 = Wait on Notification(notifier=w433, timeout in ms (-1)=w421, error in (no error)=w432) -> (notification=w431:u32, error out=w425:errorcluster)  [unwired: 1 in, 2 out]
            n133 = Merge Errors(w425, w424) -> (w426:errorcluster)
            n134 = Array Size(array=w419) -> (size(s)=w420:i32)
          }
          frame #1 {
            n135 = global read "DebugGlobal.vi" "Last Median Filter Updated"() -> (w444:string)
            n136 = global read "DebugGlobal.vi" "Camera Frame Rate (Hz)"() -> (w447:dbl)
            n137 = Quotient & Remainder(x=w462, y=w443) -> (x-y*floor(x/y)=w442:i32)  [unwired: 1 out]
            n138 = global read "DebugGlobal.vi" "Tracking Missed Frames"() -> (w445:dbl)
            n139 = global read "DebugGlobal.vi" "Camera Buffer Number"() -> (w448:u32)
            n140 = global read "DebugGlobal.vi" "Camera Missed Frames"() -> (w446:dbl)
            n141 = call <vilib>:"IMAQdx Get Image.vi"("Buffer Number Mode (Next)"=IMAQdx_Buffer_Number_Mode."Buffer Number", "error in"=w466, "Buffer Number In"=w465, "Image In"=w463, "Session In"=w464) -> ("error out"=w458:errorcluster, "Image Out"=w457:T3)  [unwired: 3 in, 2 out]
            n142 = global read "DebugGlobal.vi" "Tracking Rate (Hz)"() -> (w449:dbl)
            n143 = Index Array(array=w461, index=w442) -> (element=w460:T3)
            n144 = local write "Camera Input"(w457) -> ()
            n145 = disable-structure shown="Enabled" {
              disable-tunnel: w460 -> [w474 w475]
              disable-tunnel: w459 -> [w473 _]
              disable-tunnel: [w472 _] -> w451
              disable-tunnel: [w471 w475] -> w450
              frame Disabled {
                n146 = call "IMAQ ColorEqualize"("Image Dst"=w473, "Image Src"=w474) -> ("error out"=w472:errorcluster, "Image Dst Out"=w471:T3)  [unwired: 3 in]
              }
              frame Enabled {
              }
            }
            n147 = call "IMAQ Copy"("error in (no error)"=w458, "Image Dst"=w456, "Image Src"=w457) -> ("error out"=w455:errorcluster, "Image Dst Out"=w454:T3)  [unwired: 3 in]
            n148 = call "draw_tracking_image.vi"("error in (no error)"=w455, "Image In"=w454) -> ("error out"=w435:errorcluster, "Image Out"=w453:T3)  [unwired: 8 in]
            n149 = local write "Processed Image"(w453) -> ()
            n150 = local write "Stimulus Image"(w450) -> ()
            n151 = local read "Selected Track Index"() -> (w438:i32)
            n152 = local write "Last Median Filter Updated"(w444) -> ()
            n153 = local write "Camera Frame Rate (Hz)"(w447) -> ()
            n154 = local write "Camera Missed Frames"(w446) -> ()
            n155 = local write "Camera Buffer Number"(w448) -> ()
            n156 = local write "Tracking Rate (Hz)"(w449) -> ()
            n157 = local write "Tracking Missed Frames"(w445) -> ()
            n158 = call "active_tracks_functional_global.vi"("error in"=w435, "Operations"=ActiveTracksFunctionalGlobalOperations."ReturnAllActiveTrackIndecies") -> ("error out"=w434:errorcluster, "Active Track Indecies"=w437:i32[])  [unwired: 5 in, 3 out]
            n159 = Search 1D Array(1D array=w437, element=w438) -> (index of element=w440:i32)  [unwired: 1 in]
            n160 = Greater Or Equal To 0?(x=w440) -> (x >= 0?=w439:bool)
            n161 = case shown="False" w439 {
              tunnel: w438 -> [_ w470]
              tunnel: w437 -> [w469 _]
              tunnel: [w468 w470] -> w436
              frame False {
                n162 = Index Array(array=w469) -> (element=w468:i32)  [unwired: 1 in]
                n163 = local write "Selected Track Index"(w468) -> ()
              }
              frame True {
              }
            }
            n164 = Merge Errors(w434, w451) -> (w452:errorcluster)
          }
        }
        n165 = Tick Count (ms)() -> (millisecond timer value=w380:u32)
        n166 = local read "GUI Refresh Period (ms)"() -> (w383:u32)
        n167 = Subtract(x=w382, y=w380) -> (x-y=w381:u32)
        n168 = Max & Min(x=w381, y=w383) -> (min(x,y)=w379:u32)  [unwired: 1 out]
        n169 = Wait (ms)(milliseconds to wait=w379) -> ()  [unwired: 1 out]
        n170 = global write "DebugGlobal.vi" "GUI Refresh Period (ms)"(w379) -> ()
        n171 = Subtract(x=w380, y=w387) -> (x-y=w386:u32)
        n172 = Divide(x=w386, y=1000.0) -> (x/y=w384:dbl)
        n173 = local write "total time elapsed (s)"(w384) -> ()
        n174 = global read "DebugGlobal.vi" "Draw Stimulus Frame Rate (Hz)"() -> (w391:dbl)
        n175 = global read "DebugGlobal.vi" "Draw Stimulus Missed Frames"() -> (w392:dbl)
        n176 = global read "DebugGlobal.vi" "Projector Saving Lag (frames)"() -> (w389:i32)
        n177 = global read "DebugGlobal.vi" "median closed loop lag (ms)"() -> (w395:dbl)
        n178 = global read "DebugGlobal.vi" "Camera Saving Lag (frames)"() -> (w393:i32)
        n179 = global read "DebugGlobal.vi" "Closed Loop Lag (frames)"() -> (w394:i32)
        n180 = flat-sequence {
          frame #0 {
            n181 = global read "DebugGlobal.vi" "Debug Image"() -> (w415:T3)
            n182 = local write "Single Worm Image"(w415) -> ()
          }
          frame #1 {
            n183 = global write "DebugGlobal.vi" "Debug Image Update"(TRUE ("Debug Image Update")) -> ()
          }
        }
        n184 = global write "DebugGlobal.vi" "Debug Track Index"(w375) -> ()
        n185 = global read "DebugGlobal.vi" "Mature Tracks Count"() -> (w377:i32)
        n186 = global read "DebugGlobal.vi" "Completed Tracks #"() -> (w376:i32)
        n187 = global read "DebugGlobal.vi" "Active Tracks Count"() -> (w378:i32)
        n188 = Unbundle By Name(w406) -> ("status"=w396:bool)
        n189 = local write "median closed loop lag (ms)"(w395) -> ()
        n190 = local write "Closed Loop Lag (frames)"(w394) -> ()
        n191 = local write "Saving Lag (Camera Frames)"(w393) -> ()
        n192 = local write "Projector Saving Lag (Projector Frames)"(w389) -> ()
        n193 = local write "Draw Stimulus Frame Rate (Hz)"(w391) -> ()
        n194 = local write "Draw Stimulus Missed Frames"(w392) -> ()
        n195 = local read "stop"() -> (w405:bool)
        n196 = global read "DebugGlobal.vi" "Stop Recording"() -> (w374:bool)
        n197 = Or(x=w396, y=w405) -> (x .or. y?=w373:bool)
        n198 = Or(x=w373, y=w374) -> (x .or. y?=w390:bool)
        n199 = case shown="True" w373 {
          frame False {
          }
          frame True {
            n200 = global write "DebugGlobal.vi" "Stop Recording"(TRUE ("stop")) -> ()
            n201 = global write "DebugGlobal.vi" "Stop Reason"("GUI" ("Stop Debug")) -> ()
          }
        }
        n202 = local write "Mature Tracks Count"(w377) -> ()
        n203 = local write "Completed Tracks #"(w376) -> ()
        n204 = local write "Active Tracks Count"(w378) -> ()
      }
      n205 = call "main_image_aquisition.vi"("notifier in"=w349, "error in (no error)"=w348, "queue in"=w353, "Session In"=w352) -> ("error out"=w371:errorcluster)  [unwired: 5 in]
      n206 = call "main_save_camera_images.vi"("error in (no error)"=w348, "Median Filtered Image"=w361, "Session In"=w352, "Queue in"=w353) -> ("error out"=w370:errorcluster, "Decoded Camera Frmes"=w360:i32[])  [unwired: 6 in]
      n207 = call "main_median_filter_update.vi"("error in (no error)"=w348, "Median Filtered Image"=w351, "Spaced Out Images"=w368, "Session In"=w352) -> ("error out"=w369:errorcluster)  [unwired: 7 in]
      n208 = call "main_track.vi"("camera notifier"=w349, "error in (no error)"=w348, "tracking notifier in"=w350, "Median Filter Image"=w351, "Session In"=w352) -> ("error out"=w367:errorcluster)  [unwired: 6 in]
      n209 = call "main_save_projector_images.vi"("error in"=w348, "Array"=w355, "Queue in"=w354) -> ("error out"=w362:errorcluster)  [unwired: 8 in]
      n210 = call "main_draw_projector.vi"("camera notifier in"=w349, "projector loop queue in"=w354, "stimulus loop notifier in"=w356, "error in"=w348, "stimulus saving buffer"=w355, "ProjectorScaledImage in"=w357, "ProjectorImage in"=w358) -> ("error out"=w372:errorcluster)  [unwired: 4 in]
    }
    frame #8 {
      # "copy over the calibration obtained in the beginning"
      # "display green circle calibration image"
      n211 = global read "ParametersGlobal.vi" "Calibration Projector Dot Radius (projector pixel)"() -> (w488:i32)
      n212 = global read "ParametersGlobal.vi" "PureGreenExposureTime"() -> (w476:i32)
      n213 = Release Notifier(notifier=w504, error in (no error)=w505) -> (error out=w506:errorcluster)  [unwired: 1 in, 2 out]
      n214 = Release Queue(queue=w513, error in (no error)=w511) -> (error out=w514:errorcluster)  [unwired: 1 in, 2 out]
      n215 = global read "ParametersGlobal.vi" "Projector Calibration Points"() -> (w487:cluster{"X":dbl, "Y":dbl}[])
      n216 = Release Notifier(notifier=w512, error in (no error)=w514) -> (error out=w486:errorcluster)  [unwired: 1 in, 2 out]
      n217 = Release Queue(queue=w493, error in (no error)=w506) -> (error out=w479:errorcluster)  [unwired: 1 in, 2 out]
      n218 = call "active_tracks_functional_global.vi"("error in"=w507, "Operations"=ActiveTracksFunctionalGlobalOperations."CompleteAllActiveTracks") -> ("error out"=w510:errorcluster)  [unwired: 5 in, 4 out]
      n219 = call "initialize_projector.vi"("Green Only"=TRUE, "error in"=w479, "green exp_time_us"=w476) -> ("error out"=w478:errorcluster)  [unwired: 8 in]
      n220 = global read "ParametersGlobal.vi" "Projector Camera Calibration Original"() -> (w484:T3)
      n221 = global read "ParametersGlobal.vi" "Projector Camera Calibration Image"() -> (w483:T3)
      n222 = global read "DebugGlobal.vi" "Stop Reason"() -> (w494:string)
      n223 = call "completed_tracks_functional_gloabl.vi"("error in (no error)"=w510, 10:CompletedTracksFunctionalGlobalOperations."TrimAndReturnAllTracks") -> ("error out"=w480:errorcluster, "OutputTracks"=w481:T12[])  [unwired: 6 in, 2 out]
      n224 = call "IMAQ FillImage"("Color Pixel Value"=u32 0, "error in (no error)"=w478, "Image"=w495) -> ("error out"=w496:errorcluster, "Image Out"=w490:T3)  [unwired: 7 in]
      n225 = Array Size(array=w481) -> (size(s)=w491:i32)
      n226 = call "generate_spatial_calibration_pattern.vi"("error in (no error)"=w496, "Dot Radius (Projector Pixels)"=w488, "Points Array"=w487, "StimulusImageIn"=w490) -> ("error out"=w502:errorcluster, "StimulusImageOut"=w489:T3)  [unwired: 6 in]
      n227 = local write "Completed Tracks #"(w491) -> ()
      n228 = local write "Stop Debug"(w494) -> ()
      n229 = flat-sequence {
        tunnel: w492 -> [_]
        frame #0 {
          # "display update delay"
          n230 = Wait (ms)(milliseconds to wait=u32 1000) -> ()  [unwired: 1 out]
        }
      }
      n231 = call "IMAQ Expand"("Y Duplication Step"=2, "error in (no error)"=w502, "Image Dst"=w499, "Image Src"=w489) -> ("error out"=w500:errorcluster, "Image Dst Out"=w498:T3)  [unwired: 6 in]
      n232 = local write "Stimulus Image"(w489) -> ()
      n233 = call "IMAQ WindDraw"("Resize to Image Size? (Y)"=FALSE, "error in (no error)"=w500, "Image"=w498) -> ("error out"=w492:errorcluster)  [unwired: 7 in, 1 out]
      n234 = call "IMAQ Copy Vision Info"("error in (no error)"=w486, "Image Dst"=w484, "Image Src"=w483) -> ("error out"=w485:errorcluster)  [unwired: 6 in, 2 out]
    }
    frame #9 {
      n235 = call "snap_single_image.vi"("error in (no error)"=w542, "Session In"=w538) -> ("error out"=w540:errorcluster, "Image Out"=w539:T3)  [unwired: 8 in]
      n236 = call "calculate_deviation_from_spatial_standard.vi"("Image Src"=w539, "Background Image"=w541, "error in (no error)"=w540) -> ("Processed Image"=w533:T3, "transformation_description"=w543:dbl[], "fit least squares error (camera pixel)"=w537:dbl, "max spatial drift (mm)"=w523:dbl, "error out"=w536:errorcluster)  [unwired: 3 in]
      n237 = local write "Camera Input"(w539) -> ()
      n238 = call <vilib>:"IMAQdx Stop Acquisition.vi"("error in"=w536, "Session In"=w538) -> ("error out"=w557:errorcluster, "Session Out"=w558:T11)  [unwired: 8 in]
      n239 = call <vilib>:"IMAQdx Unconfigure Acquisition.vi"("error in"=w557, "Session In"=w558) -> ("error out"=w560:errorcluster, "Session Out"=w559:T11)  [unwired: 8 in]
      n240 = local write "Spatial Correction Fit Error (camera pixel)"(w537) -> ()
      n241 = local write "transformation_description"(w543) -> ()
      n242 = local write "Last Calibration"(w523) -> ()
      n243 = call <vilib>:"IMAQdx Close Camera.vi"("error in"=w560, "Session In"=w559) -> ("error out"=w545:errorcluster)  [unwired: 9 in]
      n244 = call "IMAQ WindClose"("Close All Windows (False)"=TRUE, "error in (no error)"=w545) -> ("error out"=w535:errorcluster)  [unwired: 4 in]
      n245 = call "check_drift_during_experiment.vi"("error in (no error)"=w535, "Processed Image"=w533, "max spatial drift since calibration (mm)"=w523) -> ("error out"=w534:errorcluster, "max spatial drift since experiment start (mm)"=w522:sgl, "Image Out"=w532:T3, "Warning needed"=w550:bool)  [unwired: 5 in]
      "Experiment Start" <- w522
      n246 = call "save_tracks_to_mat.vi"("Max Spatial Drift Since Experiment Start (mm)"=w522, "Max Spatial Drift Since Last Calibration (mm)"=w523, "DecodedCameraFrames"=w528, "error in"=w526, "Completed Tracks"=w527) -> ("error out"=w525:errorcluster, "total time elapsed (ms)"=w524:i32)  [unwired: 4 in, 1 out]
      n247 = local read "Last Experiment of the Day"() -> (w551:bool)
      n248 = local write "Processed Image"(w532) -> ()
      n249 = Merge Errors(w534, w553, w555, w556, w525, w554, w547) -> (w544:errorcluster)
      n250 = call <vilib>:"General Error Handler.vi"("error in (no error)"=w544) -> ("error out"=w552:errorcluster)  [unwired: 10 in, 4 out]
      n251 = Divide(x=w524, y=1000.0) -> (x/y=w530:dbl)
      n252 = local write "total time elapsed (s)"(w530) -> ()
      n253 = case shown="True" w551 {
        tunnel: w552 -> [w574 w576]
        tunnel: [w574 w579] -> w549
        frame False {
        }
        frame True {
          # "turn off projector"
          # "post processing"
          n254 = local read "SSH user name"() -> (w577:string)
          n255 = local read "SSH password"() -> (w578:string)
          n256 = call "turn_off_projector.vi"("error in"=w576) -> ("error out"=w575:errorcluster)  [unwired: 10 in]
          n257 = call "post_processing.vi"("error in (no error)"=w575, "SSH password"=w578, "SSH user name"=w577) -> ("error out"=w579:errorcluster)  [unwired: 8 in]
        }
      }
      n258 = Wait (ms)(milliseconds to wait=u32 5000) -> ()  [unwired: 1 out]
      n259 = case shown="True" w550 {
        tunnel: w549 -> [w562 w573]
        tunnel: [w561 w572] -> w548
        tunnel: w523 -> [_ w571]
        tunnel: w522 -> [_ w570]
        frame False {
          n260 = call "IMAQ Dispose"("All Images? (No)"=TRUE, "error in (no error)"=w562) -> ("error out"=w561:errorcluster)  [unwired: 4 in]
        }
        frame True {
          n261 = Number To Fractional String(number=w570) -> (F-format string=w566:string)  [unwired: 3 in]
          n262 = Number To Fractional String(number=w571) -> (F-format string=w568:string)  [unwired: 3 in]
          n263 = Concatenate Strings("possible miscalibration with ", w568, "mm max drift since last calibration and " ("string"), w566, "mm max drift since experiment start" ("string")) -> (w564:string)
          n264 = call "Display Message to User"("error in (no error)"=w573, "Message"=w564) -> ("error out"=w572:errorcluster)  [unwired: 8 in, 1 out]
        }
      }
    }
  }
  n265 = disable-structure shown="Disabled" {
    frame Disabled {
      n266 = call "display_active_track_snippets.vi"() -> ("Latest Active Worm Tracks"=→"Latest Active Worm Tracks":T1[])  [unwired: 3 in, 3 out]
    }
    frame Enabled {
    }
  }
  "error out" <- w66
